vi "Threshold by max & min.vi"(9 "min":dbl, 10 "max":dbl, 11 "array":dbl[](array[numeric])) -> (1 "index of min value":dbl, 2 "index of max - index of min":dbl, 3 "index of max value":dbl)   [LabVIEW 2017, in "Processing.lvlib"]
uses:
  Processing.lvlib
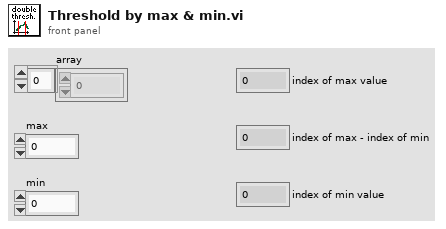
[diagram p1: front panel]
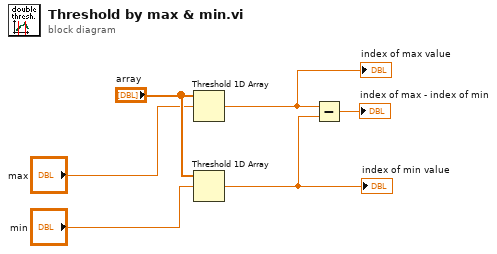
[diagram p0: block diagram]
diagram:
  n1 = Threshold 1D Array(2:"max", 3:"array") -> (0:w4:dbl)  [unwired: 1 in]
  "index of max value" <- w4
  n2 = Threshold 1D Array(2:"min", 3:"array") -> (0:w6:dbl)  [unwired: 1 in]
  "index of min value" <- w6
  n3 = Subtract(x=w4, y=w6) -> (x-y=→"index of max - index of min":dbl)
